vi "visionTester.vi"() -> ()   [LabVIEW 2016]
uses:
  <vilib>/Rock Robotics/WPI/Camera/WPI_CameraSettings Read MJPG.ctl
  <vilib>/Rock Robotics/WPI/Camera/WPI_CameraImageSize.ctl
  <vilib>/vision/NI_Vision_Development_Module.lvlib
panel:
  out "Region Reports":T1(array[cluster]) {"Mean Value" format="%.2f"; "%" format="%.2f"; "Area (calibrated)" format="%.2f"; "Maximal Value" format="%.2f"; "Minimal Value" format="%.2f"; "Standard Variation" format="%.2f"}
  out "Global Report":T2 {"Mean Value" format="%.2f"; "%" format="%.2f"; "Area (calibrated)" format="%.2f"; "Maximal Value" format="%.2f"; "Minimal Value" format="%.2f"; "Standard Variation" format="%.2f"}
  out "error out":errorcluster
  out "roiMask":T3(plugin-control)
  out "Image":T3(plugin-control)
  in  "Camera Settings":T4={"fps"=30, "compression"=30, "Image Size"=enum."320x240", "Config Shown"=FALSE}
  in  "address":string="10.te.am.11"
  in  "stop":bool
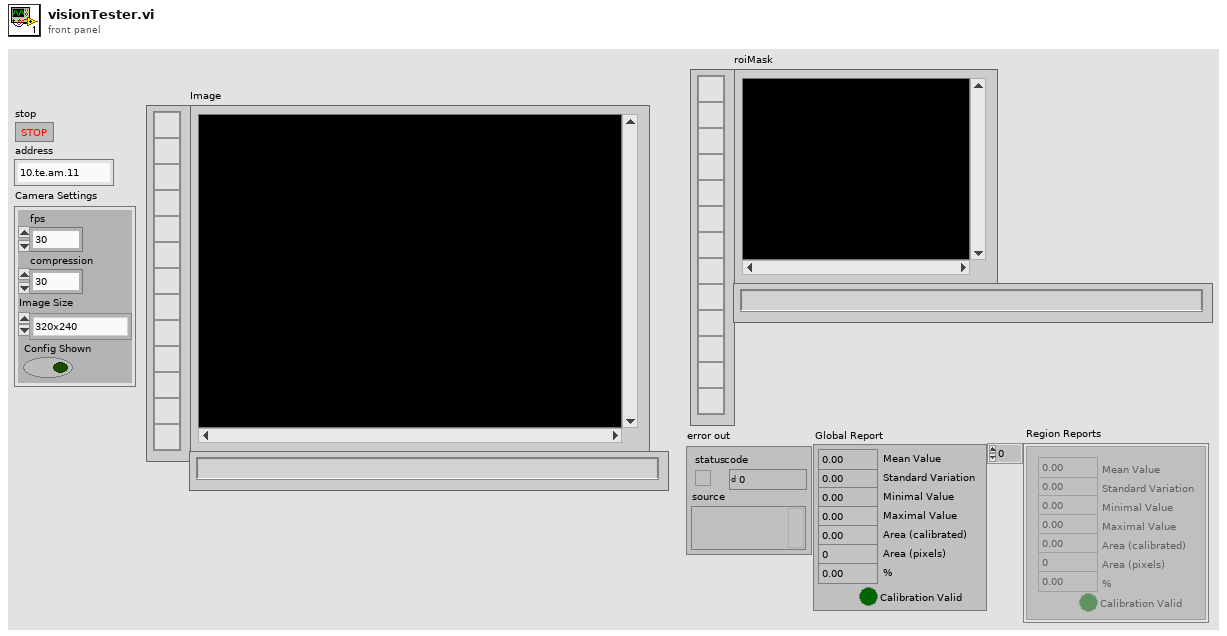
[diagram p1: front panel]
types:
  T1 = cluster{"Mean Value":sgl, "Standard Variation":sgl, "Minimal Value":sgl, "Maximal Value":sgl, "Area (calibrated)":sgl, "Area (pixels)":u32, "%":sgl, "Calibration Valid":bool}[]
  T2 = cluster{"Mean Value":sgl, "Standard Variation":sgl, "Minimal Value":sgl, "Maximal Value":sgl, "Area (calibrated)":sgl, "Area (pixels)":u32, "%":sgl, "Calibration Valid":bool}
  T3 = typedef "IMAQ Image.ctl" = refnum<image>
  T4 = typedef "WPI_CameraSettings Read MJPG.ctl" = cluster{"fps":i32, "compression":i32, "Image Size":T5, "Config Shown":bool}
  T5 = typedef "WPI_CameraImageSize.ctl" = enum16{"640x480", "320x240", "160x120", "Custom"}
  T6 = typedef "Image Type" = u32
  T7 = cluster{"Global Rectangle":i32[], "Contours":cluster{"Contour Type":u32, "ROI Type":u32, "Points":i32[]}[]}
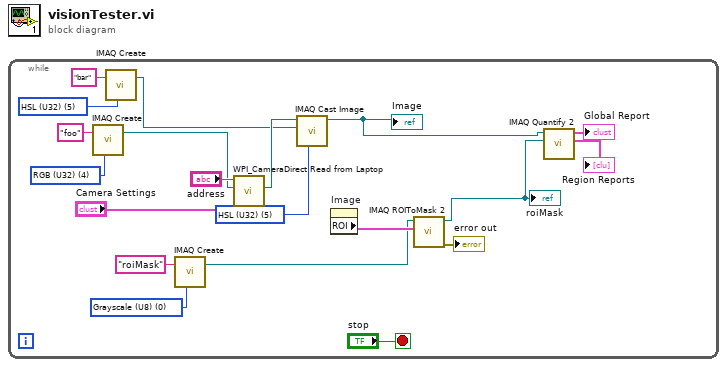
[diagram p0: block diagram]
diagram:
  n1 = while {
    stop <- "stop" stop-if-true
    w8 = T6 0 items=["Grayscale (U8)", "Grayscale (I16)", "Grayscale (SGL)", "Complex (CSG)", "RGB (U32)", "HSL (U32)", "RGB (U64)", "Grayscale (U16)"] ("Image Type")
    w10 = T6 5 items=["Grayscale (U8)", "Grayscale (I16)", "Grayscale (SGL)", "Complex (CSG)", "RGB (U32)", "HSL (U32)", "RGB (U64)", "Grayscale (U16)"] ("Image Type")
    w12 = T6 5 items=["Grayscale (U8)", "Grayscale (I16)", "Grayscale (SGL)", "Complex (CSG)", "RGB (U32)", "HSL (U32)", "RGB (U64)", "Grayscale (U16)"] ("Image Type")
    w15 = T6 4 items=["Grayscale (U8)", "Grayscale (I16)", "Grayscale (SGL)", "Complex (CSG)", "RGB (U32)", "HSL (U32)", "RGB (U64)", "Grayscale (U16)"] ("Image Type")
    n2 = call "IMAQ Create"("Image Name"="foo", "Image Type"=w15) -> ("New Image"=w16:T3)  [unwired: 3 in, 1 out]
    n3 = call "IMAQ Create"("Image Name"="bar", "Image Type"=w12) -> ("New Image"=w11:T3)  [unwired: 3 in, 1 out]
    n4 = call "IMAQ Create"("Image Name"="roiMask", "Image Type"=w8) -> ("New Image"=w6:T3)  [unwired: 3 in, 1 out]
    n5 = call <vilib>:"WPI_CameraDirect Read from Laptop.vi"("Camera Settings"="Camera Settings", "Image"=w16, "address"="address") -> ("Image Out"=w14:T3)  [unwired: 7 in, 1 out]
    n6 = call "IMAQ Cast Image"("Image Type"=w10, "Image Dst"=w11, "Image Src"=w14) -> ("Image Dst Out"=w3:T3)  [unwired: 7 in, 1 out]
    "Image" <- w3
    n7 = property on="Image" class="ImageControl"() -> ("ROI"=w9:T7)  [unwired: 2 in, 2 out]
    n8 = call "IMAQ ROIToMask 2"("ROI Descriptor"=w9, "Image"=w6) -> ("error out"=→"error out":errorcluster, "Image Out"=w4:T3)  [unwired: 7 in, 1 out]
    "roiMask" <- w4
    n9 = call "IMAQ Quantify 2"("Image Mask"=w4, "Image"=w3) -> ("Region Reports"=→"Region Reports":T1, "Global Report"=→"Global Report":T2)  [unwired: 7 in, 1 out]
  }
